vi "Write.vi"(8 "error in (no error)":errorcluster caption="entrée d'erreur (pas d'erreur)", 11 "Class UART Nodon.lvclass En entrée":refnum<class "Class UART Nodon.lvclass">) -> (0 "error out":errorcluster caption="sortie d'erreur", 3 "Class UART Nodon.lvclass En entrée":refnum<class "Class UART Nodon.lvclass">)   [LabVIEW 2020, in "Library Instrument & Equipement.lvlib" / "Library UART.lvlib" / "Class UART Nodon.lvclass"]
uses:
  Class UART Nodon.lvclass
  UART (Default)/Class UART (Default).lvclass
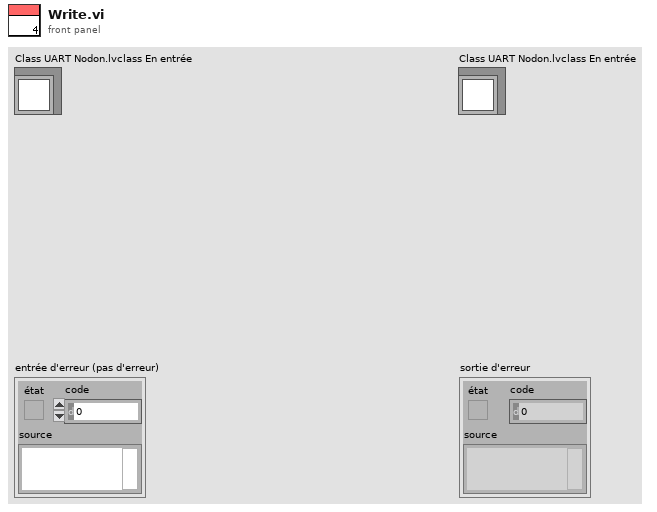
[diagram p1: front panel]
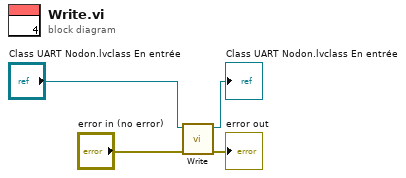
[diagram p0: block diagram]
diagram:
  n1 = call-parent "Write.vi"("error in (no error)"="error in (no error)", "Class UART (Default) en entrée"="Class UART Nodon.lvclass En entrée") -> ("error out"=→"error out":errorcluster, "Class UART (Default) en sortie"=→"Class UART Nodon.lvclass En entrée":refnum<class "Class UART Nodon.lvclass">)  [unwired: 8 in]
